vi "UHR-Fleezers Control (host) -Leonardo 04-2018 V4_fish.vi"(0 "Tab Green FB":T5(tab)=enum."Trap Control (RF)") -> ()   [LabVIEW 2014] (continued)
        n485 = Negate(x="Phase adj. (AI1)") -> (-x=w849:i16)
        n486 = Select(t=w849, s="- phase (AI1)", f="Phase adj. (AI1)") -> (s? t:f=w848:i16)
        n487 = xnode "Read/Write Control"("FPGA VI Reference In"=w852, "error in"=w851, "Phase count adjustment"=w848) -> ("FPGA VI Reference Out"=w847:T20, "error out"=w846:errorcluster)
        n488 = Or(x="- phase (AI1)", y="+ phase (AI1)") -> (x .or. y?=w843:bool)
        n489 = xnode "Read/Write Control"("FPGA VI Reference In"=w847, "error in"=w846, "+ phase"=w843) -> ("error out"=w842:errorcluster)  [unwired: 1 out]
      }
      event "Signals to Plot": Double Click {
        w855 = u32 9868950 ("Color Box")
        n490 = event-data() -> ("Row"=w857:i32)  [unwired: 9 out]
        n491 = property on="All Signals" class="WFChart (strict)"("Active Plot"=w857) -> (error out=w868:errorcluster)  [unwired: 2 in, 1 out]
        n492 = property on="All Signals" class="WFChart (strict)" props=["Plot", "Visible?", "Plot", "Plot Color"](error in=w868) -> (error out=w867:errorcluster, "Plot.Visible?"=w866:bool)  [unwired: 1 in, 2 out]
        n493 = Select(t=FALSE ("Plot.Visible"), s=w866, f=TRUE ("Plot.Visible")) -> (s? t:f=w861:bool)
        n494 = property on="All Signals" class="WFChart (strict)"(error in=w867, "Plot.Visible?"=w861) -> (error out=w863:errorcluster)  [unwired: 1 in, 1 out]
        n495 = property on="All Signals" class="WFChart (strict)"(error in=w863) -> (error out=w858:errorcluster, "Plot.Plot Color"=w862:u32)  [unwired: 1 in, 1 out]
        n496 = property on="Signals to Plot" class="LstBox (strict)"(error in=w858, "Active Row"=w857) -> (error out=w856:errorcluster)  [unwired: 1 in, 1 out]
        n497 = Select(t=w862, s=w861, f=u32 0) -> (s? t:f=w859:u32)
        n498 = property on="Signals to Plot" class="LstBox (strict)"(error in=w856, "CellFontColor"=w859, "SelColor"=w855, "CellBG"=w855, "CellFontSize"=u32 20 ("Active Row:Cell Font:Size"), "CellFontBold"=TRUE ("Active Row:Cell Font:Bold")) -> ()  [unwired: 1 in, 2 out]
      }
      event "Dynamic Force FB": Value Change {
        n499 = event-data() -> ()  [unwired: 7 out]
        n500 = xnode "Read/Write Control"("FPGA VI Reference In"=w870, "Dynamic Force FB (Ronen)"="Dynamic Force FB") -> ()  [unwired: 1 in, 2 out]
      }
      event "BD 1 Frequency 1 (MHz)", "BD 1 Frequency 2 (MHz)", "BD 1 Frequency 3 (MHz)", "BD 2 Frequency 1 (MHz)", "BD 2 Frequency 2 (MHz)", "BD 2 Frequency 3 (MHz)", "Trap Delta (MHz)": Value Change {
        # "anytime one of the frequencies is changed, write it to the RF board UNLESS Set 2 is being oscillated. The oscillation\nscript writes the frequencies to the RF board."
        n501 = event-data() -> ("CtlRef"=w873:refnum<vi>)  [unwired: 6 out]
        n502 = control-ref of="Trap Delta (MHz)"() -> (w872:refnum<vi>)
        n503 = Equal?(x=w872, y=w873) -> (x = y?=w871:bool)
        n504 = case shown="False" "Oscillate Set 2" {
          tunnel: w876 -> [w897 _]
          tunnel: [w896 w909] -> w875
          tunnel: w874 -> [w895 w909]
          tunnel: w871 -> [w882 _]
          frame False {
            n505 = case shown="True" "Symmetric manual \ntrap motion" {
              tunnel: ["T2 for asymmetric\n(MHz)" w908] -> w883
              tunnel: "Trap Delta (MHz)" -> [w902 w907]
              tunnel: [w901 w904] -> w879
              frame False {
                n506 = Subtract(x="T2 for asymmetric\n(MHz)", y=w902) -> (x-y=w901:dbl)
              }
              frame True {
                n507 = Divide(x=w907, y=2) -> (x/y=w905:dbl)
                n508 = Subtract(x="Middle freq for \nsymmetric (MHz)", y=w905) -> (x-y=w904:dbl)
                n509 = Add(x="Middle freq for \nsymmetric (MHz)", y=w905) -> (x+y=w908:dbl)
              }
            }
            n510 = local read "BD 1 Frequency 2 (MHz)"() -> (w884:dbl)
            n511 = local write "BD 1 Frequency 1 (MHz)"(w879) -> ()
            n512 = Select(t=w883, s=w882, f=w884) -> (s? t:f=w881:dbl)
            n513 = local read "Y RF Frequency Limits (MHz)"() -> (w885:T16)
            n514 = local read "X RF Frequency Limits (MHz)"() -> (w886:T16)
            n515 = local read "BD 1 Frequency 3 (MHz)"() -> (w898:dbl)
            n516 = local write "BD 1 Frequency 2 (MHz)"(w881) -> ()
            n517 = local read "BD 2 Frequency 1 (MHz)"() -> (w889:dbl)
            n518 = local read "BD 2 Frequency 2 (MHz)"() -> (w888:dbl)
            n519 = local read "BD 2 Frequency 3 (MHz)"() -> (w899:dbl)
            n520 = call "set RF board frequency - interlace.vi"("Board 2 Frequency Limits"=w885, "Board 1 Frequency Limits"=w886, "error in"=w895, "FPGA VI Reference In"=w897, "Board 2 Frequency 3 (MHz)"=w899, "Board 1 Frequency 3 (MHz)"=w898, "Board 2 Frequency 2 (MHz)"=w888, "Board 2 Frequency 1 (MHz)"=w889, "Board 1 Frequency 2 (MHz)"=w881, "Board 1 Frequency 1  (MHz)"=w879) -> ("error out"=w896:errorcluster)  [unwired: 1 out]
            n521 = Subtract(x=w889, y=w888) -> (x-y=w893:dbl)
            n522 = Subtract(x=w881, y=w879) -> (x-y=w894:dbl)
            n523 = Square(x=w893) -> (x^2=w891:dbl)
            n524 = Square(x=w894) -> (x^2=w892:dbl)
            n525 = Add(x=w892, y=w891) -> (x+y=w890:dbl)
            n526 = Square Root(x=w890) -> (sqrt(x)=w887:dbl)
            n527 = local write "Trap Delta (MHz)"(w887) -> ()
            n528 = property on="Initial delta (MHz)" class="DigNum (strict)"("Val(Sgnl)"=w887) -> ()  [unwired: 2 in, 2 out]
          }
          frame True {
          }
        }
      }
      event "Round T1 X": Value Change {
        n529 = event-data() -> ()  [unwired: 7 out]
        n530 = local read "BD 1 Frequency 1 (MHz)"() -> (w912:dbl)
        n531 = Round To Nearest(number=w912) -> (nearest integer value=w911:dbl)
        n532 = property on="BD 1 Frequency 1 (MHz)" class="DigNum (strict)"("Val(Sgnl)"=w911) -> ()  [unwired: 2 in, 2 out]
      }
      event "Round T2 X": Value Change {
        n533 = event-data() -> ()  [unwired: 7 out]
        n534 = local read "BD 1 Frequency 2 (MHz)"() -> (w914:dbl)
        n535 = Round To Nearest(number=w914) -> (nearest integer value=w913:dbl)
        n536 = property on="BD 1 Frequency 2 (MHz)" class="DigNum (strict)"("Val(Sgnl)"=w913) -> ()  [unwired: 2 in, 2 out]
      }
      event "Stop All": Value Change {
        n537 = event-data() -> ()  [unwired: 7 out]
        n538 = call "hamilton_controller.vi"("action"=T21."DISCONNECT") -> ()  [unwired: 10 in, 1 out]
        n539 = local read "Stop All"() -> (w917:bool)
      }
      event "Delayed Interlace Start": Value Change {
        n540 = event-data() -> ()  [unwired: 7 out]
        n541 = flat-sequence {
          frame #0 {
            n542 = Multiply(x="Delay to Interlace (s)", y=1000.0) -> (x*y=w920:dbl)
            n543 = Wait (ms)(milliseconds to wait=w920) -> ()  [unwired: 1 out]
          }
          frame #1 {
            n544 = property on="Green laser mode" class="RadioBtnsControl (strict)"("Val(Sgnl)"=enum32{"Laser ON", "Laser OFF", "Interlace"}."Interlace" ("Value (Signaling)")) -> ()  [unwired: 2 in, 2 out]
          }
        }
      }
      event "BD 1 Amplitude 1 (%)", "BD 1 Amplitude 2 (%)", "BD 1 Amplitude 3 (%)", "BD 2 Amplitude 1 (%)", "BD 2 Amplitude 2 (%)", "BD 2 Amplitude 3 (%)", "Trap 1 ON", "Trap 2 ON", "Trap 3 ON", "Feedback On/Off", "All FB On/Off": Value Change {
        w944 = i16 1 ("f")
        n545 = event-data() -> ()  [unwired: 7 out]
        n546 = local write "Trap 1 (ON/OFF)"("Trap 1 ON") -> ()
        n547 = local write "Trap 2 (ON/OFF)"("Trap 2 ON") -> ()
        n548 = Boolean To (0,1)(Boolean="Trap 3 ON") -> (0, 1=w945:i16)
        n549 = Boolean To (0,1)(Boolean="Trap 1 ON") -> (0, 1=w946:i16)
        n550 = Boolean To (0,1)(Boolean="Trap 2 ON") -> (0, 1=w947:i16)
        n551 = Select(t=w947, s="Trap ON/OFF X or Y Amp?", f=w944) -> (s? t:f=w942:i16)
        n552 = Select(t=w946, s="Trap ON/OFF X or Y Amp?", f=w944) -> (s? t:f=w943:i16)
        n553 = Select(t=w945, s="Trap ON/OFF X or Y Amp?", f=w944) -> (s? t:f=w941:i16)
        n554 = Select(t=w944, s="Trap ON/OFF X or Y Amp?", f=w947) -> (s? t:f=w939:i16)
        n555 = Select(t=w944, s="Trap ON/OFF X or Y Amp?", f=w946) -> (s? t:f=w940:i16)
        n556 = Select(t=w944, s="Trap ON/OFF X or Y Amp?", f=w945) -> (s? t:f=w938:i16)
        n557 = And(x="All FB On/Off", y="Feedback On/Off") -> (x .and. y?=w936:cluster{"Set 1":bool, "Set 2":bool})
        n558 = local read "BD 1 Amplitude 1 (%)"() -> (w956:dbl)
        n559 = local read "BD 1 Amplitude 2 (%)"() -> (w955:dbl)
        n560 = local read "BD 1 Amplitude 3 (%)"() -> (w954:dbl)
        n561 = Unbundle By Name(w936) -> ("Set 1"=w932:bool, "Set 2"=w929:bool)
        n562 = local read "Y RF Amplitude Limits (%)"() -> (w925:T16)
        n563 = local read "X RF Amplitude Limits (%)"() -> (w926:T16)
        n564 = local read "BD 2 Amplitude 1 (%)"() -> (w957:dbl)
        n565 = local read "BD 2 Amplitude 2 (%)"() -> (w958:dbl)
        n566 = local read "BD 2 Amplitude 3 (%)"() -> (w959:dbl)
        n567 = And(x="Trap 2 ON", y=w929) -> (x .and. y?=w927:bool)
        n568 = And(x="Trap 1 ON", y=w932) -> (x .and. y?=w930:bool)
        n569 = Multiply(x=w943, y=w956) -> (x*y=w951:dbl)
        n570 = Multiply(x=w955, y=w942) -> (x*y=w949:dbl)
        n571 = Multiply(x=w954, y=w941) -> (x*y=w950:dbl)
        n572 = Multiply(x=w957, y=w940) -> (x*y=w960:dbl)
        n573 = Multiply(x=w958, y=w939) -> (x*y=w961:dbl)
        n574 = Multiply(x=w959, y=w938) -> (x*y=w962:dbl)
        n575 = call "set RF board amplitude - interlace.vi"("Board 2 Amplitude Limits"=w925, "Board 1 Amplitude Limits"=w926, "error in"=w952, "FPGA VI Reference In"=w953, "Board 2 Amplitude 3 (%)"=w962, "Board 1 Amplitude 3 (%)"=w950, "Board 2 Amplitude 2 (%)"=w961, "Board 2 Amplitude 1 (%)"=w960, "Board 1 Amplitude 2 (%)"=w949, "Board 1 Amplitude 1 (%)"=w951) -> ("error out"=w934:errorcluster, "FPGA VI Reference Out"=w935:T20)
        n576 = xnode "Read/Write Control"("FPGA VI Reference In"=w935, "error in"=w934, "FB On/Off Set 1"=w930, "FB On/Off Set 2"=w927) -> ("error out"=w933:errorcluster)  [unwired: 1 out]
        n577 = case shown="True" "All FB On/Off" {
          frame False {
          }
          frame True {
            n578 = local write "Feedback overload"(FALSE) -> ()
          }
        }
      }
      event "Load parameters": Value Change {
        n579 = event-data() -> ()  [unwired: 7 out]
        n580 = property on="Saved AOD Raster Scan Parameter Sets" class="Arr (strict)"() -> ("Index Values"=w974:u32[])  [unwired: 2 in, 2 out]
        n581 = Index Array(array=w974, index=0) -> (element=w971:u32)
        n582 = local write "Load parameters"(FALSE ("Load parameters")) -> ()
        n583 = Index Array(array="Saved AOD Raster Scan Parameter Sets", index=w971) -> (element=w970:T31)
        n584 = Unbundle By Name(w970) -> ("Scan Range AOD (nm) 2"=w969:dbl, "Step Size AOD (nm) 2"=w968:dbl, "Scan Speed AOD (nm/s) 2"=w967:dbl, "Number of scans (AOD) 2"=w966:u16)
        n585 = flat-sequence {
          tunnel: w969 -> [w977]
          tunnel: w968 -> [w976]
          tunnel: w967 -> [w975]
          tunnel: w966 -> [w978]
          frame #0 {
            n586 = local write "Scan Speed (nm/s)"(w975) -> ()
            n587 = local write "Scan Range (nm)"(w977) -> ()
            n588 = local write "Step Size (nm)"(w976) -> ()
          }
          frame #1 {
            n589 = property on="Number of F/B Scans (AOD)" class="DigNum (strict)"("Val(Sgnl)"=w978) -> ()  [unwired: 2 in, 2 out]
          }
        }
      }
      event "Trap 1 (ON/OFF)", "Trap 2 (ON/OFF)": Value Change {
        n590 = event-data() -> ()  [unwired: 7 out]
        n591 = property on="Trap 2 ON" class="Bool (strict)"("Val(Sgnl)"="Trap 2 (ON/OFF)") -> ()  [unwired: 2 in, 2 out]
        n592 = property on="Trap 1 ON" class="Bool (strict)"("Val(Sgnl)"="Trap 1 (ON/OFF)") -> ()  [unwired: 2 in, 2 out]
      }
      event "DIO count 1 (ticks)", "DIO count 2 (ticks)", "DIO count 3 (ticks)", "Interlace", "Number Interlace Sets", "Not-Interlacing Set": Value Change {
        n593 = event-data() -> ()  [unwired: 7 out]
        n594 = local read "DIO count 3 (ticks)"() -> (w991:u32)
        n595 = local read "DIO count 1 (ticks)"() -> (w993:u32)
        n596 = local read "DIO count 2 (ticks)"() -> (w992:u32)
        n597 = To Unsigned Byte Integer(number="Not-Interlacing Set") -> (unsigned 8bit integer=w982:u8)
        n598 = Add(x=w982, y=u8 1) -> (x+y=w986:u8)
        n599 = xnode "Read/Write Control"("FPGA VI Reference In"=w997, "error in"=w995, "DIO count 1 (ticks)"=w993, "DIO count 2 (ticks)"=w992, "DIO count 3 (ticks)"=w991, "Interlace ON/OFF"="Interlace", "Number Interlace Cycles"="Number Interlace Sets", "Interlace Off Parameters"=w986) -> ("error out"=w996:errorcluster)  [unwired: 1 out]
        n600 = Build Array(w993, w992, w991) -> (w984:u32[])
        n601 = Split 1D Array(array=w984, index="Number Interlace Sets") -> (first subarray=w994:u32[])  [unwired: 1 out]
        n602 = Index Array(array=w984, index=w982) -> (element=w983:u32)
        n603 = Add Array Elements(numeric array=w994) -> (sum=w988:u32)
        n604 = Select(t=w988, s="Interlace", f=w983) -> (s? t:f=→"Total Counts (ticks)":u32)
      }
      event "Reset Feedback": Value Change {
        n605 = event-data() -> ()  [unwired: 7 out]
        n606 = Unbundle By Name("Reset Feedback") -> ("Set 1"=w1001:bool, "Set 2"=w1000:bool)
        n607 = xnode "Read/Write Control"("FPGA VI Reference In"=w1003, "error in"=w998, "FB Reset Set 1"=w1001, "FB Reset Set 2"=w1000) -> ("error out"=w999:errorcluster)  [unwired: 1 out]
      }
      event "PID gains": Value Change {
        n608 = event-data() -> ()  [unwired: 7 out]
        n609 = local read "PID gains"() -> (w1004:T10)
        n610 = xnode "Read/Write Control"("FPGA VI Reference In"=w1007, "error in"=w1005, "FB Gains"=w1004) -> ("error out"=w1006:errorcluster)  [unwired: 1 out]
      }
      event "AI2 to Setpoint", "Trap Intensity\nSetpoints (V)": Value Change {
        n611 = event-data() -> ()  [unwired: 7 out]
        n612 = xnode "Read/Write Control"("FPGA VI Reference In"=w1012, "error in"=w1008) -> ("FPGA VI Reference Out"=w1011:T20, "error out"=w1010:errorcluster, "AI2 Y Sum Set 1"=w1019:i16, "AI2 Y Sum Set 2"=w1018:i16)
        n613 = Cluster To Array(cluster="AI2 to Setpoint") -> (array=w1022:bool[])
        n614 = local read "AI2 (V)"() -> (w1020:cluster{"Set 1":dbl, "Set 2":dbl})
        n615 = Or Array Elements(Boolean array=w1022) -> (logical OR=w1023:bool)
        n616 = Bundle By Name(cluster=w1020, "Set 1"=w1019, "Set 2"=w1018) -> (w1017:cluster{"Set 1":dbl, "Set 2":dbl})
        n617 = Divide(x=w1017, y=3276.7) -> (x/y=w1016:cluster{"Set 1":dbl, "Set 2":dbl})
        "AI2 (V)" <- w1016
        n618 = case shown="True" w1023 {
          tunnel: [w1026 w1043] -> w1015
          tunnel: "AI2 to Setpoint" -> [_ w1039]
          tunnel: "Trap Intensity\nSetpoints (V)" -> [w1027 w1042]
          tunnel: w1016 -> [_ w1036]
          frame False {
            n619 = Multiply(x=3276.7, y=w1027) -> (x*y=w1028:cluster{"Set 1":dbl, "Set 2":dbl})
            n620 = To Word Integer(number=w1028) -> (16bit integer=w1026:cluster{"Set 1":i16, "Set 2":i16})
          }
          frame True {
            n621 = Unbundle By Name(w1036) -> ("Set 1"=w1035:dbl, "Set 2"=w1034:dbl)
            n622 = Unbundle By Name(w1042) -> ("Set 1"=w1041:dbl, "Set 2"=w1040:dbl)
            n623 = Unbundle By Name(w1039) -> ("Set 1"=w1038:bool, "Set 2"=w1037:bool)
            n624 = Select(t=w1035, s=w1038, f=w1041) -> (s? t:f=w1033:dbl)
            n625 = Select(t=w1034, s=w1037, f=w1040) -> (s? t:f=w1032:dbl)
            n626 = Bundle By Name(cluster=w1042, "Set 1"=w1033, "Set 2"=w1032) -> (w1030:cluster{"Set 1":dbl, "Set 2":dbl})
            n627 = local write "Trap Intensity\nSetpoints (V)"(w1030) -> ()
            n628 = Multiply(x=3276.7, y=w1030) -> (x*y=w1031:cluster{"Set 1":dbl, "Set 2":dbl})
            n629 = To Word Integer(number=w1031) -> (16bit integer=w1043:cluster{"Set 1":i16, "Set 2":i16})
          }
        }
        n630 = Unbundle By Name(w1015) -> ("Set 1"=w1014:i16, "Set 2"=w1013:i16)
        n631 = xnode "Read/Write Control"("FPGA VI Reference In"=w1011, "error in"=w1010, "FB Setpoint Set 1"=w1014, "FB Setpoint Set 2"=w1013) -> ("error out"=w1009:errorcluster)  [unwired: 1 out]
      }
      event "Invert GI": Value Change {
        n632 = event-data() -> ()  [unwired: 7 out]
        n633 = xnode "Read/Write Control"("FPGA VI Reference In"=w1048, "error in"=w1046, "Invert GI"="Invert GI", "Invert GI 2"="Invert GI") -> ("error out"=w1047:errorcluster)  [unwired: 1 out]
      }
      event "Green FB Setpoint (mV)", "Green FB Gains", "Green FB On/Off", "Current When FB OFF (%)", "Green int current ON count adj": Value Change {
        n634 = event-data() -> ()  [unwired: 7 out]
        n635 = local read "Green FB Setpoint (mV)"() -> (w1055:dbl)
        n636 = local read "Current When FB OFF (%)"() -> (w1058:dbl)
        n637 = Multiply(x=w1055, y=3.2767) -> (x*y=w1054:dbl)
        n638 = Multiply(x=w1058, y=655.35) -> (x*y=w1059:dbl)
        n639 = To Unsigned Word Integer(number=w1059) -> (unsigned 16bit integer=w1057:u16)
        n640 = local read "Green int current ON count adj"() -> (w1062:u32)
        n641 = local read "Green FB Gains"() -> (w1061:T10)
        n642 = local read "Green Laser ON/Interlacing"() -> (w1052:bool)
        n643 = local read "Green laser mode"() -> (w1051:enum32{"Laser ON", "Laser OFF", "Interlace"})
        n644 = local read "Green FB On/Off"() -> (w1063:bool)
        n645 = Equal?(x=w1051, y=enum32{"Laser ON", "Laser OFF", "Interlace"}."Interlace") -> (x = y?=w1049:bool)
        n646 = Compound Arithmetic op=AND(w1049, w1063, w1052) -> (w1053:bool)
        n647 = xnode "Read/Write Control"("FPGA VI Reference In"=w1066, "error in"=w1065, "Green FB Setpoint"=w1054, "Green FB On/Off"=w1053, "Current Out"=w1057, "Green int current ON count adj"=w1062, "Green FB Gains"=w1061) -> ("error out"=w1064:errorcluster)  [unwired: 1 out]
      }
      event "Green laser mode", "Green Laser ON/Interlacing": Value Change {
        n648 = event-data() -> ()  [unwired: 7 out]
        n649 = case shown="True" "Green Laser ON/Interlacing" {
          tunnel: "Green laser mode" -> [_ w1080]
          tunnel: [enum32{"Laser ON", "Laser OFF", "Interlace"}."Laser OFF" ("Green laser mode") w1080] -> w1068
          tunnel: [FALSE w1076] -> w1067
          frame False {
          }
          frame True {
            n650 = local read "Green FB On/Off"() -> (w1077:bool)
            n651 = Equal?(x=w1080, y=enum32{"Laser ON", "Laser OFF", "Interlace"}."Interlace") -> (x = y?=w1078:bool)
            n652 = And(x=w1078, y=w1077) -> (x .and. y?=w1076:bool)
          }
        }
        n653 = xnode "Read/Write Control"("FPGA VI Reference In"=w1073, "error in"=w1071, "Operating Mode"=w1068, "Operating Mode 2"=w1068, "Green FB On/Off"=w1067) -> ("error out"=w1072:errorcluster)  [unwired: 1 out]
      }
      event "- phase (APD 1 Gate)", "+ phase (APD 1 Gate)": Value Change {
        n654 = event-data() -> ()  [unwired: 7 out]
        n655 = local read "Phase Adj. (APD 1 Gate)"() -> (w1081:i16)
        n656 = Negate(x=w1081) -> (-x=w1089:i16)
        n657 = Select(t=w1089, s="- phase (APD 1 Gate)", f=w1081) -> (s? t:f=w1088:i16)
        n658 = Or(x="- phase (APD 1 Gate)", y="+ phase (APD 1 Gate)") -> (x .or. y?=w1084:bool)
        n659 = xnode "Read/Write Control"("FPGA VI Reference In"=w1091, "error in"=w1090, "Phase count adjustment (APD 1 Gate)"=w1088) -> ("FPGA VI Reference Out"=w1086:T20, "error out"=w1087:errorcluster)
        n660 = xnode "Read/Write Control"("FPGA VI Reference In"=w1086, "error in"=w1087, "+ phase (APD 1 Gate)"=w1084) -> ("error out"=w1085:errorcluster)  [unwired: 1 out]
      }
      event "+ phase (APD 2 Gate)", "- phase (APD 2 Gate)": Value Change {
        n661 = event-data() -> ()  [unwired: 7 out]
        n662 = local read "Phase Adj. (APD 2 Gate)"() -> (w1092:i16)
        n663 = Negate(x=w1092) -> (-x=w1100:i16)
        n664 = Select(t=w1100, s="- phase (APD 2 Gate)", f=w1092) -> (s? t:f=w1099:i16)
        n665 = Or(x="- phase (APD 2 Gate)", y="+ phase (APD 2 Gate)") -> (x .or. y?=w1095:bool)
        n666 = xnode "Read/Write Control"("FPGA VI Reference In"=w1102, "error in"=w1101, "Phase count adjustment (APD 2 Gate)"=w1099) -> ("FPGA VI Reference Out"=w1097:T20, "error out"=w1098:errorcluster)
        n667 = xnode "Read/Write Control"("FPGA VI Reference In"=w1097, "error in"=w1098, "+ phase (APD 2 Gate)"=w1095) -> ("error out"=w1096:errorcluster)  [unwired: 1 out]
      }
      event "Phase Adj. (APD Acq)", "+ phase (APD Acq)", "- phase (APD Acq)": Value Change {
        n668 = event-data() -> ()  [unwired: 7 out]
        n669 = local read "Phase Adj. (APD Acq)"() -> (w1105:i16)
        n670 = Negate(x=w1105) -> (-x=w1111:i16)
        n671 = Select(t=w1111, s="+ phase (APD Acq)", f=w1105) -> (s? t:f=w1110:i16)
        n672 = Or(x="+ phase (APD Acq)", y="- phase (APD Acq)") -> (x .or. y?=w1106:bool)
        n673 = xnode "Read/Write Control"("FPGA VI Reference In"=w1113, "error in"=w1112, "Phase Count Adjustment (APD Acq)"=w1110) -> ("FPGA VI Reference Out"=w1108:T20, "error out"=w1109:errorcluster)
        n674 = xnode "Read/Write Control"("FPGA VI Reference In"=w1108, "error in"=w1109, "+ phase (APD Acq)"=w1106) -> ("error out"=w1107:errorcluster)  [unwired: 1 out]
      }
      event "Phase adj. (GI)", "+ phase (GI)", "- phase (GI)": Value Change {
        n675 = event-data() -> ()  [unwired: 7 out]
        n676 = Negate(x="Phase adj. (GI)") -> (-x=w1122:i16)
        n677 = Select(t=w1122, s="+ phase (GI)", f="Phase adj. (GI)") -> (s? t:f=w1121:i16)
        n678 = Or(x="+ phase (GI)", y="- phase (GI)") -> (x .or. y?=w1117:bool)
        n679 = xnode "Read/Write Control"("FPGA VI Reference In"=w1124, "error in"=w1123, "Phase count adjustment (GI)"=w1121) -> ("FPGA VI Reference Out"=w1119:T20, "error out"=w1120:errorcluster)
        n680 = xnode "Read/Write Control"("FPGA VI Reference In"=w1119, "error in"=w1120, "+ phase (GI)"=w1117) -> ("error out"=w1118:errorcluster)  [unwired: 1 out]
      }
      event "Phase adj. (GI) 2", "+ phase (GI) 2", "- phase (GI) 2": Value Change {
        n681 = event-data() -> ()  [unwired: 7 out]
        n682 = Negate(x="Phase adj. (GI) 2") -> (-x=w1133:i16)
        n683 = Select(t=w1133, s="+ phase (GI) 2", f="Phase adj. (GI) 2") -> (s? t:f=w1132:i16)
        n684 = Or(x="+ phase (GI) 2", y="- phase (GI) 2") -> (x .or. y?=w1128:bool)
        n685 = xnode "Read/Write Control"("FPGA VI Reference In"=w1135, "error in"=w1134, "Phase count adjustment (GI) 2"=w1132) -> ("FPGA VI Reference Out"=w1130:T20, "error out"=w1131:errorcluster)
        n686 = xnode "Read/Write Control"("FPGA VI Reference In"=w1130, "error in"=w1131, "+ phase (GI) 2"=w1128) -> ("error out"=w1129:errorcluster)  [unwired: 1 out]
      }
      event "Phase adj. (Green FB)", "- phase (Green FB)", "+ phase (Green FB)": Value Change {
        n687 = event-data() -> ()  [unwired: 7 out]
        n688 = Negate(x="Phase adj. (Green FB)") -> (-x=w1144:i16)
        n689 = Select(t=w1144, s="+ phase (Green FB)", f="Phase adj. (Green FB)") -> (s? t:f=w1143:i16)
        n690 = Or(x="+ phase (Green FB)", y="- phase (Green FB)") -> (x .or. y?=w1139:bool)
        n691 = xnode "Read/Write Control"("FPGA VI Reference In"=w1146, "error in"=w1145, "Phase count adjustment (Green FB)"=w1143) -> ("FPGA VI Reference Out"=w1141:T20, "error out"=w1142:errorcluster)
        n692 = xnode "Read/Write Control"("FPGA VI Reference In"=w1141, "error in"=w1142, "+ phase (Green FB)"=w1139) -> ("error out"=w1140:errorcluster)  [unwired: 1 out]
      }
      event "Invert APD Gate", "APD Gate ON Count", "APD Gate OFF Count", "APD Gate", "APD Integration Time (s)", "APD 1 AO Mult.", "APD 2 AO Mult.": Value Change {
        n693 = event-data() -> ()  [unwired: 7 out]
        n694 = local read "APD Integration Time (s)"() -> (w1147:dbl)
        n695 = local read "APD Gate ON Count"() -> (w1160:u32)
        n696 = local read "APD Gate OFF Count"() -> (w1159:u32)
        n697 = local read "Invert APD Gate"() -> (w1161:bool)
        n698 = local read "APD Gate"() -> (w1158:enum32{"ON", "OFF", "Interlace"})
        n699 = Multiply(x=w1147, y=40000000.0) -> (x*y=w1156:dbl)
        n700 = Reciprocal(x=w1147) -> (1/x=→"APD Acq Rate (Hz)":dbl)
        n701 = To Unsigned Long Integer(number=w1156) -> (unsigned 32bit integer=w1155:u32)
        n702 = local read "DMA Update Period (s)"() -> (w1148:dbl)
        n703 = Divide(x=w1148, y=w1147) -> (x/y=w1151:dbl)
        n704 = local read "APD 1 AO Mult."() -> (w1153:i16)
        n705 = local read "APD 2 AO Mult."() -> (w1152:i16)
        n706 = Multiply(x=2.0, y=w1151) -> (x*y=w1150:dbl)
        n707 = local write "APD Samples/FIFO Acq."(w1151) -> ()
        n708 = local write "APD Elements/DMA read"(w1150) -> ()
        n709 = xnode "Read/Write Control"("FPGA VI Reference In"=w1164, "error in"=w1163, "Invert APD Gate"=w1161, "APD Gate ON Count"=w1160, "APD Gate OFF Count"=w1159, "APD Acq Rate Count"=w1155, "APD Gate Operating Mode"=w1158, "APD 1 AO scale factor"=w1153, "APD 2 AO scale factor"=w1152) -> ("error out"=w1162:errorcluster)  [unwired: 1 out]
      }
      event "GI Frequency, ON count", "Green FB Count", "GI Frequency, OFF count": Value Change {
        n710 = event-data() -> ()  [unwired: 7 out]
        n711 = xnode "Read/Write Control"("FPGA VI Reference In"=w1170, "error in"=w1168, "Green interlace ON count"="GI Frequency, ON count", "Green interlace OFF count"="GI Frequency, OFF count", "Green interlace ON count 2"="GI Frequency, ON count", "Green interlace OFF count 2"="GI Frequency, OFF count", "Green FB Count"="Green FB Count") -> ("error out"=w1169:errorcluster)  [unwired: 1 out]
      }
      event "Number of F/B Scans (AOD)", "Scan Speed (nm/s)", "Scan BD", "Initial delta (MHz)", "Step Size (nm)", "Scan Range (nm)": Value Change {
        w1232 = 123.0  # AOM cal (nm/MHz)
        n712 = event-data() -> ()  [unwired: 7 out]
        n713 = local read "BD 1 Frequency 1 (MHz)"() -> (w1215:dbl)
        n714 = local read "AOM X Cal (nm/MHz)"() -> (w1207:dbl)
        n715 = local read "X RF Frequency Limits (MHz)"() -> (w1219:T16)
        n716 = local read "Y RF Frequency Limits (MHz)"() -> (w1216:T16)
        n717 = local read "BD 2 Frequency 1 (MHz)"() -> (w1221:dbl)
        n718 = Negate(x="Scan Range (nm)") -> (-x=w1185:dbl)
        n719 = Divide(x=w1185, y=w1207) -> (x/y=w1189:dbl)
        n720 = Select(t=w1219, s="Scan BD", f=w1216) -> (s? t:f=w1218:T16)
        n721 = Select(t=w1215, s="Scan BD", f=w1221) -> (s? t:f=w1220:dbl)
        n722 = Unbundle By Name(w1218) -> ("Maximum"=w1227:dbl, "Minimum"=w1226:dbl)
        n723 = Add(x=w1189, y=w1220) -> (x+y=w1224:dbl)
        n724 = Divide(x=w1185, y="Step Size (nm)") -> (x/y=w1204:dbl)
        n725 = Divide(x="Step Size (nm)", y=w1207) -> (x/y=w1213:dbl)
        n726 = Absolute Value(x=w1204) -> (abs(x)=w1188:dbl)
        n727 = Sign(1:w1185) -> (0:w1186:dbl)
        n728 = In Range and Coerce(upper limit=w1227, x=w1224, lower limit=w1226) -> (coerced(x)=w1223:dbl, In Range?=w1225:bool)
        n729 = To Unsigned Quad Integer(1:w1188) -> (0:w1203:u64)
        "Scan steps (AOD)" <- w1203
        n730 = call "IR AOM freq to word.vi"("Frequency In (MHz)"=w1213) -> ("Frequency Word Out (double)"=w1210:dbl)
        n731 = Multiply(x=w1186, y=w1210) -> (x*y=w1187:dbl)
        n732 = Subtract(x=w1224, y=w1223) -> (x-y=w1222:dbl)
        n733 = To Quad Integer(1:w1187) -> (0:w1209:i64)
        "Incr. int (AOD)" <- w1209
        n734 = Subtract(x=w1189, y=w1222) -> (x-y=w1208:dbl)
        "Scan Range (MHz)" <- w1208
        n735 = Select(t=w1189, s=w1225, f=w1208) -> (s? t:f=w1228:dbl)
        n736 = Multiply(x=w1208, y=w1207) -> (x*y=w1206:dbl)
        n737 = Decrement(x=w1203) -> (x-1=w1256:u64)
        n738 = Negate(x=w1206) -> (-x=w1202:dbl)
        n739 = local write "Scan Range (nm)"(w1202) -> ()
        n740 = Divide(x=w1228, y=w1256) -> (x/y=w1212:dbl)
        "Scan Increment (MHz)" <- w1212
        n741 = call "IR AOM freq to word.vi"("Frequency In (MHz)"=w1212) -> ("Frequency Word Out (double)"=w1211:dbl)
        n742 = Divide(x="Step Size (nm)", y="Scan Speed (nm/s)") -> (x/y=w1199:dbl)
        n743 = To Quad Integer(1:w1211) -> ()  [unwired: 1 out]
        n744 = local read "Number Interlace Sets"() -> (w1183:u8)
        n745 = local read "AI Count (ticks)"() -> (w1184:u32)
        n746 = local read "Total Counts (ticks)"() -> (w1182:u32)
        n747 = local read "# Samples/trap"() -> (w1214:u32)
        n748 = Multiply(x=w1184, y=w1183) -> (x*y=w1181:u32)
        n749 = Divide(x=w1182, y=w1181) -> (x/y=w1180:dbl)
        n750 = Select(t=w1215, s="Scan BD", f=w1221) -> (s? t:f=w1253:dbl)
        "Initial freq. (MHz)" <- w1253
        n751 = Add(x=w1228, y=w1253) -> (x+y=→"Final freq. (MHz)":dbl)
        n752 = Divide(x=w1182, y=40000000.0) -> (x/y=w1198:dbl)
        n753 = Divide(x=w1199, y=w1198) -> (x/y=w1197:dbl)
        n754 = To Unsigned Quad Integer(1:w1197) -> (0:w1172:u64)
        n755 = Quotient & Remainder(x=w1172, y=u64 2) -> (x-y*floor(x/y)=w1176:u64)  [unwired: 1 out]
        n756 = Equal?(x=w1176, y=u64 0) -> (x = y?=w1174:bool)
        n757 = Decrement(x=w1172) -> (x-1=w1173:u64)
        n758 = Select(t=w1172, s=w1174, f=w1173) -> (s? t:f=w1171:u64)
        "Cycles/step (AOD)" <- w1171
        n759 = xnode "Read/Write Control"("FPGA VI Reference In"=w1264, "error in"=w1263, "Scan steps"=w1203, "Number of scans"="Number of F/B Scans (AOD)", "Cycles per step"=w1171, "Scan freq.  increment"=w1209, "Scan BD"="Scan BD") -> ("error out"=w1262:errorcluster)  [unwired: 1 out]
        n760 = Multiply(x=w1203, y=w1171) -> (x*y=w1257:u64)
        n761 = Multiply(x=w1257, y=u64 2) -> (x*y=w1179:u64)
        n762 = Multiply(x=w1180, y=w1179) -> (x*y=w1178:dbl)
        "Data points/scan (f/b)" <- w1178
        n763 = Multiply(x=w1178, y="Number of F/B Scans (AOD)") -> (x*y=w1260:dbl)
        "Data points/scans" <- w1260
        n764 = Divide(x=w1260, y=w1214) -> (x/y=→"N sets should be saved":dbl)
        n765 = Multiply(x=w1257, y=w1198) -> (x*y=w1196:dbl)
        "Time/Scan (s) (AOD)" <- w1196
        n766 = Select(t=w1228, s="Scan BD", f=0.0) -> (s? t:f=w1254:dbl)
        n767 = Select(t=0.0, s="Scan BD", f=w1228) -> (s? t:f=w1250:dbl)
        n768 = local read "BD 2 Frequency 2 (MHz)"() -> (w1246:dbl)
        n769 = local read "BD 1 Frequency 2 (MHz)"() -> (w1249:dbl)
        n770 = Add(x=w1250, y=w1221) -> (x+y=w1247:dbl)
        n771 = Add(x=w1215, y=w1254) -> (x+y=w1248:dbl)
        n772 = Multiply(x=w1196, y=2.0) -> (x*y=w1195:dbl)
        n773 = Multiply(x=w1195, y="Number of F/B Scans (AOD)") -> (x*y=w1192:dbl)
        n774 = Divide(x=w1192, y=60.0) -> (x/y=→"Time to Finish All (min)":dbl)
        n775 = Add(x="Trap 2 Bead Size (nm)", y="Trap 1 Bead Size (nm)") -> (x+y=w1236:dbl)
        n776 = local read "Initial delta (MHz)"() -> (w1233:dbl)
        n777 = Divide(x=w1236, y=2.0) -> (x/y=w1230:dbl)
        n778 = Subtract(x=w1247, y=w1246) -> (x-y=w1244:dbl)
        n779 = Subtract(x=w1248, y=w1249) -> (x-y=w1245:dbl)
        n780 = Square(x=w1244) -> (x^2=w1243:dbl)
        n781 = Square(x=w1245) -> (x^2=w1242:dbl)
        n782 = Add(x=w1242, y=w1243) -> (x+y=w1241:dbl)
        n783 = Square Root(x=w1241) -> (sqrt(x)=w1240:dbl)
        "Final delta (MHz)" <- w1240
        n784 = Multiply(x=w1232, y=w1240) -> (x*y=w1239:dbl)
        n785 = Multiply(x=w1233, y=w1232) -> (x*y=w1231:dbl)
        n786 = Subtract(x=w1231, y=w1230) -> (x-y=→"Initial sep (nm)":dbl)
        n787 = Subtract(x=w1239, y=w1230) -> (x-y=→"Final sep (nm)":dbl)
      }
      event "Raster Scanning...": Value Change {
        n788 = event-data() -> ("NewVal"=w1265:bool)  [unwired: 6 out]
        n789 = case shown="True" w1265 {
          frame False {
          }
          frame True {
            n790 = property on="BD 1 Frequency 1 (MHz)" class="DigNum (strict)"("Val(Sgnl)"=65.0 ("Value (Signaling)")) -> ()  [unwired: 2 in, 2 out]
          }
        }
      }
      event "Phase increment trap 1", "Swap F1 and F2", "Freq switch delay", "Amp switch delay", "Phase increment trap 2", "RF phase reset before cycles", "Phase offset method": Value Change {
        n791 = event-data() -> ()  [unwired: 7 out]
        n792 = local read "Amp switch delay"() -> (w1271:u16)
        n793 = local read "Phase increment trap 1"() -> (w1270:fxp<+/-,64,32>)
        n794 = local read "Freq switch delay"() -> (w1273:u16)
        n795 = local read "Phase increment trap 2"() -> (w1269:fxp<+/-,64,32>)
        n796 = local read "RF phase reset before cycles"() -> (w1268:bool)
        n797 = local read "Swap F1 and F2"() -> (w1272:bool)
        n798 = local read "Phase offset method"() -> (w1267:u8)
        n799 = xnode "Read/Write Control"("FPGA VI Reference In"=w1276, "error in"=w1275, "BD 1 Delay (ticks)"=w1273, "Swap F1 and F2"=w1272, "Amp switch delay"=w1271, "Phase Trap 1"=w1270, "Phase Trap 2"=w1269, "RF phase reset before cycles"=w1268, "Phase offset method"=w1267) -> ("error out"=w1274:errorcluster)  [unwired: 1 out]
      }
      event "Scan steps (MCL)", "Number of scans (MCL)", "Scan Range (V)\n(of steps)", "2D or 1D Scan", "N APD Samp/step", "Fast Scan Dir", "Continuous MCL Scanning", "Scan lines (y)": Value Change {
        w1278 = 32767.0 ("y")
        n800 = event-data() -> ()  [unwired: 7 out]
        n801 = Select(t="Scan lines (y)", s="2D or 1D Scan", f="Number of scans (MCL)") -> (s? t:f=w1283:u64)
        n802 = Decrement(x="Scan steps (MCL)") -> (x-1=w1299:u64)
        n803 = Divide(x="Scan Range (V)\n(of steps)", y=w1299) -> (x/y=w1298:dbl)
        "Desired Scan Incr (V)" <- w1298
        n804 = local read "APD Integration Time (s)"() -> (w1291:dbl)
        n805 = Multiply(x=w1298, y=w1278) -> (x*y=w1307:dbl)
        n806 = Divide(x=w1307, y=10.0) -> (x/y=w1297:dbl)
        "Desired incr (int)" <- w1297
        n807 = local read "Update Count (MCL)"() -> (w1303:u32)
        n808 = Round Toward -Infinity(1:w1297) -> (0:w1306:dbl)
        n809 = To Word Integer(number=w1306) -> (16bit integer=w1281:i16)
        "Actual Incr. int (MCL)" <- w1281
        n810 = Multiply(x=w1291, y=40000000.0) -> (x*y=w1304:dbl)
        n811 = Divide(x=w1304, y=w1303) -> (x/y=w1302:dbl)
        n812 = Multiply(x=i16 10, y=w1281) -> (x*y=w1279:i16)
        n813 = Multiply(x="N APD Samp/step", y=w1302) -> (x*y=w1301:dbl)
        "Cycles/step (MCL)" <- w1301
        n814 = Divide(x=w1279, y=w1278) -> (x/y=→"Actual MCL Inc (V)":dbl)
        n815 = Multiply(x="N APD Samp/step", y="Scan steps (MCL)") -> (x*y=w1293:dbl)
        n816 = local read "APD Samples/FIFO Acq."() -> (w1290:dbl)
        n817 = Multiply(x=w1293, y=u64 2) -> (x*y=w1292:dbl)
        "Data points/scan (f+b)" <- w1292
        n818 = Multiply(x=w1292, y=w1283) -> (x*y=w1310:dbl)
        "Data points/scans (MCL)" <- w1310
        n819 = Multiply(x=w1291, y=w1292) -> (x*y=w1284:dbl)
        "Time/f+b scan (s) (MCL)" <- w1284
        n820 = Divide(x=w1310, y=w1290) -> (x/y=→"N sets should be saved (MCL)":dbl)
        n821 = Multiply(x=w1284, y=w1283) -> (x*y=→"Total Time (s)":dbl)
        n822 = Not(x="Fast Scan Dir") -> (.not. x?=w1288:bool)
        n823 = xnode "Read/Write Control"("FPGA VI Reference In"=w1314, "error in"=w1313, "Scan steps (MCL)"="Scan steps (MCL)", "Number of scans (MCL)"=w1283, "Cycles per step (MCL)"=w1301, "Scan freq.  increment (MCL)"=w1281, "1D or 2D Scan?"="2D or 1D Scan", "MCL Scan Axis"=w1288, "Cont. Scan (MCL)"="Continuous MCL Scanning") -> ("error out"=w1312:errorcluster)  [unwired: 1 out]
      }
      event "Read Cal": Value Change {
        w1351 = 1000.0 ("y")
        w1339 = T30."big-endian, network order" ("byte order (0:big-endian, network order)")
        w1340 = -1 ("count (1)")
        n824 = event-data() -> ()  [unwired: 7 out]
        n825 = local read "Save file name"() -> (w1369:path)
        n826 = local write "Read Cal"(FALSE ("Read Cal")) -> ()
        n827 = Strip Path(path=w1369) -> (stripped path=w1368:path)  [unwired: 1 out]
        n828 = Path To String(path=w1368) -> (string=w1349:string)
        n829 = Concatenate Strings(w1349, "\\current.off" ("string")) -> (w1347:string)
        n830 = Concatenate Strings(w1349, "\\current.cal" ("string")) -> (w1366:string)
        n831 = local read "Scale intensities"() -> (w1319:bool)
        n832 = String To Path(string=w1366) -> (path=w1365:path)
        n833 = String To Path(string=w1347) -> (path=w1346:path)
        n834 = Open/Create/Replace File(file path (use dialog)=w1365, operation (0:open)=T24."open", access (0:read/write)=enum16{"read/write", "read-only", "write-only"}."read-only") -> (refnum out=w1372:refnum<file>, error out=w1361:errorcluster)  [unwired: 1 in, 3 out]
        n835 = Deny Access(4:w1361, 7:w1372) -> (0:w1360:errorcluster, 3:w1364:refnum<file>)  [unwired: 1 out]
        n836 = Open/Create/Replace File(file path (use dialog)=w1346, operation (0:open)=T24."open", access (0:read/write)=enum16{"read/write", "read-only", "write-only"}."read-only") -> (refnum out=w1343:refnum<file>)  [unwired: 1 in, 4 out]
        n837 = Deny Access(7:w1343) -> (3:w1341:refnum<file>)  [unwired: 1 in, 2 out]
        n838 = Read from Binary File(5:0.0, 8:w1360, 9:w1339, 10:w1340, 11:w1364) -> (0:w1359:errorcluster, 2:w1357:dbl[], 3:w1362:refnum<file>)  [unwired: 2 out]
        n839 = Array To Cluster(array=w1357) -> (cluster=w1356:T32)
        n840 = Unbundle(w1356) -> ("[0]"=w1330:dbl, "[1]"=w1329:dbl, "[2]"=w1316:dbl, "[3]"=w1318:dbl, "[4]"=w1355:dbl, "[5]"=w1354:dbl)
        n841 = case "Cal is OK if you load a cal with scale intensities on - Alex 081418" shown="True" w1319 {
          tunnel: w1318 -> [w1374 w1377]
          tunnel: [w1374 w1376] -> w1317
          tunnel: w1316 -> [w1373 w1379]
          tunnel: [w1373 w1378] -> w1315
          frame False {
          }
          frame True {
            n842 = local read "Scale factor"() -> (w1375:dbl)
            n843 = Multiply(x=w1377, y=w1375) -> (x*y=w1376:dbl)
            n844 = Multiply(x=w1379, y=w1375) -> (x*y=w1378:dbl)
          }
        }
        n845 = Close File(refnum=w1362, error in=w1359) -> (error out=→"Read cal error":errorcluster)  [unwired: 1 out]
        n846 = Multiply(x=w1354, y=w1351) -> (x*y=w1352:dbl)
        n847 = local write "T2 kappa_x (pN/nm)"(w1317) -> ()
        n848 = local write "T1 kappa_x (pN/nm)"(w1315) -> ()
        n849 = local write "T1 alpha_x (nm/V)"(w1330) -> ()
        n850 = local write "T2 alpha_x (nm/V)"(w1329) -> ()
        n851 = Read from Binary File(5:0.0, 9:w1339, 10:w1340, 11:w1341) -> (2:w1335:dbl[], 3:w1338:refnum<file>)  [unwired: 1 in, 3 out]
        n852 = Multiply(x=w1355, y=w1351) -> (x*y=w1353:dbl)
        n853 = local write "T1 offset_x (mV)"(w1353) -> ()
        n854 = local write "T2 offset_x (mV)"(w1352) -> ()
        n855 = Close File(refnum=w1338) -> ()  [unwired: 1 in, 2 out]
        n856 = Array Subset(array=w1335, index=3) -> (w1333:dbl[])  [unwired: 1 in]
        n857 = Index Array(array=w1335, index=0) -> (element=→"Offset file step size":dbl)
        n858 = Multiply(x=w1330, y=w1316) -> (x*y=w1327:dbl)
        n859 = Multiply(x=w1329, y=w1318) -> (x*y=w1328:dbl)
        n860 = Divide(x=w1328, y=w1327) -> (x/y=w1321:dbl)
        n861 = Decimate 1D Array(w1333) -> (w1325:dbl[], w1326:dbl[])  [unwired: 1 out]
        n862 = disable-structure "Removed B factor to improve position FB -Alex 081418 2of3" shown="Enabled" {
          disable-tunnel: w1321 -> [w1380 _]
          disable-tunnel: [w1380 1.0] -> w1320
          frame Disabled {
          }
          frame Enabled {
          }
        }
        n863 = Bundle By Name(cluster="Offset Values", "Trap 1X offset"=w1325, "Trap 2X offset"=w1326) -> (w1331:T14)
        n864 = Multiply(x=w1326, y=w1320) -> (x*y=w1324:dbl[])
        n865 = Subtract(x=w1325, y=w1324) -> (x-y=w1323:dbl[])
        n866 = local write "Offset Values"(w1331) -> ()
        n867 = case shown="True" "Auto read offset\ncorrection" {
          tunnel: w1323 -> [_ w1382]
          frame False {
          }
          frame True {
            n868 = property on="Setpoint offset\nCorrection values" class="Arr (strict)"("Val(Sgnl)"=w1382) -> ()  [unwired: 2 in, 2 out]
          }
        }
        n869 = property on="B factor" class="DigNum (strict)"("Val(Sgnl)"=w1320) -> ()  [unwired: 2 in, 2 out]
      }
      event "Symmetric Raster/Feedback?": Value Change {
        n870 = event-data() -> ()  [unwired: 7 out]
        n871 = xnode "Read/Write Control"("FPGA VI Reference In"=w1384, "Symmetric FB/Raster"="Symmetric Raster/Feedback?") -> ()  [unwired: 1 in, 2 out]
      }
      event "Abort MCL Scan": Value Change {
        n872 = event-data() -> ()  [unwired: 7 out]
        n873 = local write "MCL Scanning"(FALSE ("MCL Scanning")) -> ()
        n874 = xnode "Read/Write Control"("FPGA VI Reference In"=w1389, "error in"=w1388, "Abort scan (MCL)"="Abort MCL Scan") -> ("error out"=w1387:errorcluster)  [unwired: 1 out]
      }
      event "Update Count (MCL)": Value Change {
        n875 = event-data() -> ()  [unwired: 7 out]
        n876 = xnode "Read/Write Control"("FPGA VI Reference In"=w1393, "error in"=w1392, "MCL count"="Update Count (MCL)") -> ("error out"=w1391:errorcluster)  [unwired: 1 out]
      }
      event "Phase adjust (MCL)", "+ phase (MCL)", "- phase (MCL)": Value Change {
        n877 = event-data() -> ()  [unwired: 7 out]
        n878 = Negate(x="Phase adjust (MCL)") -> (-x=w1402:i16)
        n879 = Select(t=w1402, s="- phase (MCL)", f="Phase adjust (MCL)") -> (s? t:f=w1400:i16)
        n880 = Or(x="- phase (MCL)", y="+ phase (MCL)") -> (x .or. y?=w1395:bool)
        n881 = xnode "Read/Write Control"("FPGA VI Reference In"=w1404, "error in"=w1403, "Phase count adjustment (MCL)"=w1400) -> ("FPGA VI Reference Out"=w1396:T20, "error out"=w1397:errorcluster)
        n882 = xnode "Read/Write Control"("FPGA VI Reference In"=w1396, "error in"=w1397, "+ phase (MCL)"=w1395) -> ("error out"=w1394:errorcluster)  [unwired: 1 out]
      }
      event "Abort AOD Scan": Value Change {
        n883 = event-data() -> ()  [unwired: 7 out]
        n884 = flat-sequence {
          tunnel: w1409 -> [w1416]
          tunnel: w1408 -> [w1415]
          tunnel: [w1414] -> w1406
          tunnel: [w1410] -> w1405
          tunnel: [w1429] -> w1407
          tunnel: w1406 -> [w1429]
          tunnel: w1405 -> [w1428]
          frame #0 {
            n885 = local read "Save scans"() -> (w1412:bool)
            n886 = xnode "Read/Write Control"("FPGA VI Reference In"=w1416, "error in"=w1415, "Abort scan"="Abort AOD Scan") -> ("FPGA VI Reference Out"=w1410:T20, "error out"=w1414:errorcluster)
            n887 = local write "Raster Scanning..."(FALSE) -> ()
            n888 = case shown="True" w1412 {
              frame False {
              }
              frame True {
                n889 = local write "Stop Saving"(TRUE) -> ()
              }
            }
          }
          frame #1 {
            n890 = xnode "Read/Write Control"("FPGA VI Reference In"=w1428) -> ("BD1 Frequency Out 1"=w1419:u64)  [unwired: 1 in, 2 out]
            n891 = To Double Precision Float(number=w1419) -> (double precision float=w1425:dbl)
            n892 = Multiply(x=49125000.0, y=6.0) -> (x*y=w1424:dbl)
            n893 = Multiply(x=w1425, y=w1424) -> (x*y=w1422:dbl)
            n894 = Scale By Power Of 2(n=-48, x=w1422) -> (x*2^n=w1421:dbl)
            n895 = Divide(x=w1421, y=1000000.0) -> (x/y=w1418:dbl)
            n896 = property on="BD 1 Frequency 1 (MHz)" class="DigNum (strict)"("Val(Sgnl)"=w1418) -> ()  [unwired: 2 in, 2 out]
          }
        }
      }
      event "Continuous AOD Scanning": Value Change {
        n897 = event-data() -> ()  [unwired: 7 out]
        n898 = xnode "Read/Write Control"("FPGA VI Reference In"=w1433, "error in"=w1432, "Cont. Scan"="Continuous AOD Scanning") -> ("error out"=w1431:errorcluster)  [unwired: 1 out]
      }
      event "Index": Value Change {
        n899 = event-data() -> ()  [unwired: 7 out]
        n900 = call "Create new save file.vi"("Insert"="", "Ext"=".dat" ("string"), "Index In"="Index") -> ("Path Out"=→"Save file name":path, "Index Out"=w1434:dbl)
        "Save index" <- w1434
        n901 = local write "Index"(w1434) -> ()
      }
      event "AO1", "AO2": Value Change {
        w1449 = 10.0 ("y")
        w1448 = 32767.0 ("y")
        n902 = event-data() -> ()  [unwired: 7 out]
        n903 = local read "AO2"() -> (w1447:dbl)
        n904 = local read "AO1"() -> (w1444:dbl)
        n905 = Multiply(x=w1444, y=w1448) -> (x*y=w1443:dbl)
        n906 = Multiply(x=w1447, y=w1448) -> (x*y=w1446:dbl)
        n907 = Divide(x=w1443, y=w1449) -> (x/y=w1442:dbl)
        n908 = Divide(x=w1446, y=w1449) -> (x/y=w1445:dbl)
        n909 = To Word Integer(number=w1442) -> (16bit integer=w1450:i16)
        n910 = To Word Integer(number=w1445) -> (16bit integer=w1451:i16)
        n911 = xnode "Read/Write Control"("FPGA VI Reference In"=w1441, "error in"=w1440, "AO1 (Y)"=w1450, "AO2 (X)"=w1451) -> ("error out"=w1439:errorcluster)  [unwired: 1 out]
      }
      event "Inject Top:": Value Change {
        n912 = event-data() -> ()  [unwired: 7 out]
        n913 = disable-structure shown="Enabled" {
          disable-tunnel: "Inject Top:" -> [w1453 w1493]
          frame Disabled {
            n914 = local read "Chemyx Syringe Pump Serial Port"() -> (w1454:refnum<visa-resource-name>)
            n915 = local read "Pump write delay (ms)"() -> (w1455:dbl)
            n916 = case shown="True" w1453 {
              tunnel: w1455 -> [w1461 w1475]
              tunnel: w1454 -> [w1458 w1474]
              frame False {
                n917 = flat-sequence {
                  tunnel: w1458 -> [w1462]
                  tunnel: [w1462] -> w1459
                  tunnel: w1461 -> [_]
                  tunnel: [w1465] -> w1460
                  tunnel: w1459 -> [w1465]
                  tunnel: w1460 -> [w1466]
                  tunnel: [w1466] -> w1456
                  tunnel: [w1468] -> w1457
                  tunnel: w1456 -> [w1468]
                  tunnel: w1457 -> [w1470]
                  frame #0 {
                    n918 = call "Write to pump.vi"("string"="enter pump1", "VISA resource name"=w1462) -> ()  [unwired: 1 out]
                  }
                  frame #1 {
                    n919 = Wait (ms)(milliseconds to wait="Pump pause delay (ms)") -> ()  [unwired: 1 out]
                  }
                  frame #2 {
                    n920 = call "Write to pump.vi"("string"="stop", "VISA resource name"=w1466) -> ()  [unwired: 1 out]
                  }
                  frame #3 {
                    n921 = Wait (ms)(milliseconds to wait=u32 500) -> ()  [unwired: 1 out]
                  }
                  frame #4 {
                    n922 = call "Write to pump.vi"("string"="stop", "VISA resource name"=w1470) -> ()  [unwired: 1 out]
                  }
                }
              }
              frame True {
                n923 = flat-sequence {
                  tunnel: w1474 -> [w1484]
                  tunnel: w1475 -> [w1479]
                  tunnel: w1475 -> [w1486]
                  tunnel: w1474 -> [w1487]
                  tunnel: [w1487] -> w1472
                  tunnel: [w1489] -> w1473
                  tunnel: w1472 -> [w1489]
                  tunnel: w1473 -> [w1491]
                  frame #0 {
                    n924 = local read "All Pump Parameters"() -> (w1478:T6)
                    n925 = Unbundle By Name(w1478) -> ("Pump 1"=w1485:T33)
                    n926 = call "Set pump parameters.vi"("Pump write delay (ms)"=w1479, "Volume (uL)"="Ch 2 Inject Volume (uL)", "Rate (uL/h)"="Ch 1 Inject Rate (ul/h)", "Units"=4.0, "Pump #"=1.0, "Pump Parameters In"=w1485, "VISA resource name"=w1484) -> ("Pump Parameters Out"=w1477:T33)  [unwired: 3 in]
                    n927 = Bundle By Name(cluster=w1478, "Pump 1"=w1477) -> (w1476:T6)
                    n928 = local write "All Pump Parameters"(w1476) -> ()
                  }
                  frame #1 {
                    n929 = Wait (ms)(milliseconds to wait=w1486) -> ()  [unwired: 1 out]
                  }
                  frame #2 {
                    n930 = call "Write to pump.vi"("string"="start", "VISA resource name"=w1487) -> ()  [unwired: 1 out]
                  }
                  frame #3 {
                    n931 = Wait (ms)(milliseconds to wait=u32 500) -> ()  [unwired: 1 out]
                  }
                  frame #4 {
                    n932 = call "Write to pump.vi"("string"="start", "VISA resource name"=w1491) -> ()  [unwired: 1 out]
                  }
                }
              }
            }
          }
          frame Enabled {
            n933 = call "hamilton_controller.vi"("Open?"=w1493, "valve"=enum16{"A", "B", "C", "D", "ALL"}."B", "action"=T21."MOVE VALVE") -> ()  [unwired: 8 in, 1 out]
          }
        }
      }
      event "Main:": Value Change {
        n934 = event-data() -> ()  [unwired: 7 out]
        n935 = disable-structure shown="Enabled" {
          disable-tunnel: "Main:" -> [_ w1537]
          frame Disabled {
            n936 = local read "Pump write delay (ms)"() -> (w1498:dbl)
            n937 = case shown="False" w1499 {
              tunnel: w1498 -> [w1505 w1519]
              tunnel: "Chemyx Syringe Pump Serial Port" -> [w1502 w1518]
              frame False {
                n938 = flat-sequence {
                  tunnel: w1502 -> [w1506]
                  tunnel: [w1506] -> w1503
                  tunnel: w1505 -> [_]
                  tunnel: [w1509] -> w1504
                  tunnel: w1503 -> [w1509]
                  tunnel: w1504 -> [w1510]
                  tunnel: [w1510] -> w1500
                  tunnel: [w1512] -> w1501
                  tunnel: w1500 -> [w1512]
                  tunnel: w1501 -> [w1514]
                  frame #0 {
                    n939 = call "Write to pump.vi"("string"="enter pump3", "VISA resource name"=w1506) -> ()  [unwired: 1 out]
                  }
                  frame #1 {
                    n940 = local read "Pump pause delay (ms)"() -> (w1508:u32)
                    n941 = Wait (ms)(milliseconds to wait=w1508) -> ()  [unwired: 1 out]
                  }
                  frame #2 {
                    n942 = call "Write to pump.vi"("string"="stop", "VISA resource name"=w1510) -> ()  [unwired: 1 out]
                  }
                  frame #3 {
                    n943 = Wait (ms)(milliseconds to wait=u32 0) -> ()  [unwired: 1 out]
                  }
                  frame #4 {
                    n944 = call "Write to pump.vi"("string"="stop", "VISA resource name"=w1514) -> ()  [unwired: 1 out]
                  }
                }
              }
              frame True {
                n945 = flat-sequence {
                  tunnel: w1518 -> [w1528]
                  tunnel: w1519 -> [w1523]
                  tunnel: w1519 -> [w1530]
                  tunnel: w1518 -> [w1531]
                  tunnel: [w1531] -> w1516
                  tunnel: [w1534] -> w1517
                  tunnel: w1516 -> [w1534]
                  tunnel: w1517 -> [w1535]
                  frame #0 {
                    n946 = local read "All Pump Parameters"() -> (w1522:T6)
                    n947 = Unbundle By Name(w1522) -> ("Pump 3"=w1529:T33)
                    n948 = call "Set pump parameters.vi"("Pump write delay (ms)"=w1523, "Volume (uL)"="Ch 3 Inject Volume (uL)", "Rate (uL/h)"="Ch 3 Inject Rate (ul/h)", "Units"=4.0, "Pump #"=3.0, "Pump Parameters In"=w1529, "VISA resource name"=w1528) -> ("Pump Parameters Out"=w1521:T33)  [unwired: 3 in]
                    n949 = Bundle By Name(cluster=w1522, "Pump 3"=w1521) -> (w1520:T6)
                    n950 = local write "All Pump Parameters"(w1520) -> ()
                  }
                  frame #1 {
                    n951 = Wait (ms)(milliseconds to wait=w1530) -> ()  [unwired: 1 out]
                  }
                  frame #2 {
                    n952 = call "Write to pump.vi"("string"="start", "VISA resource name"=w1531) -> ()  [unwired: 1 out]
                  }
                  frame #3 {
                    n953 = Wait (ms)(milliseconds to wait=u32 500) -> ()  [unwired: 1 out]
                  }
                  frame #4 {
                    n954 = call "Write to pump.vi"("string"="start", "VISA resource name"=w1535) -> ()  [unwired: 1 out]
                  }
                }
